vi "functiontest.vi"() -> ()   [LabVIEW 2017]
uses:
  <vilib>/regexp/Match Regular Expression.xnode
panel:
  out "trimmed string":string
  out "Commands out 2":string
  out "Commands out":string
  in  "Commands in":string
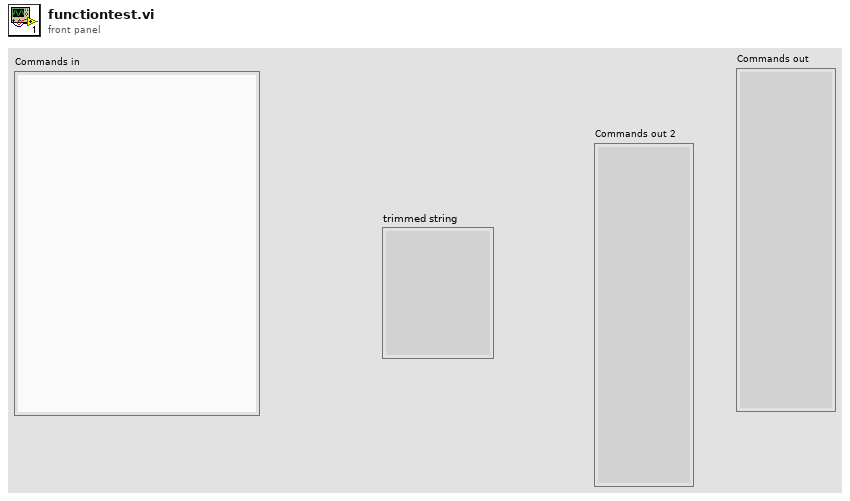
[diagram p1: front panel]
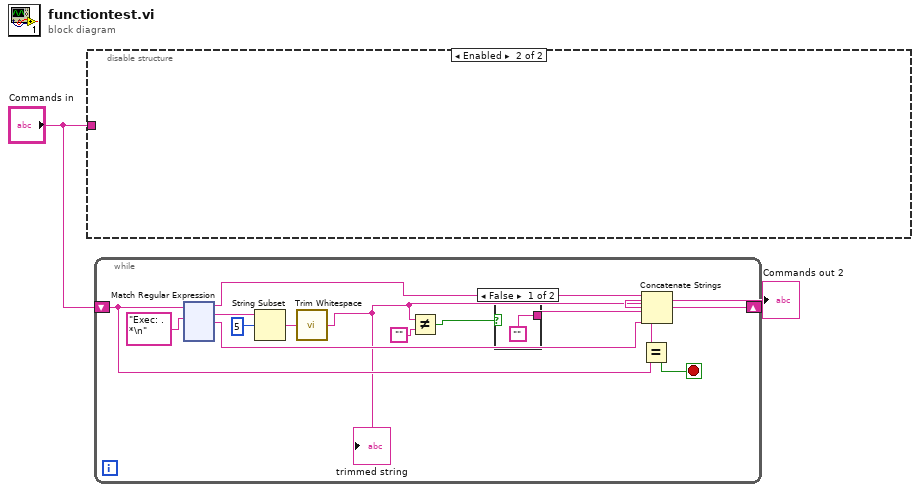
[diagram p0: block diagram]
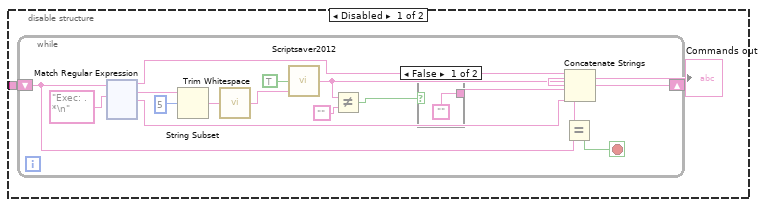
[diagram p2: hidden frame]
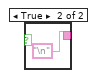
[diagram p3: hidden frame]
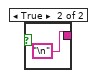
[diagram p4: hidden frame]
diagram:
  n1 = disable-structure shown="Enabled" {
    disable-tunnel: "Commands in" -> [w3 _]
    frame Disabled {
      n2 = while {
        shift-right: [w10] -> w4
        shift-left: w3 -> [w9]
        stop <- w8 stop-if-true
        n3 = xnode "Match Regular Expression"("input string"=w9, "regular expression"="Exec: .*\n") -> ("before match"=w15:string, "whole match"=w18:string, "after match"=w12:string)  [unwired: 4 in, 2 out]
        n4 = String Subset(string=w18, offset (0)=5) -> (substring=w14:string)  [unwired: 1 in]
        n5 = call <vilib>:"Trim Whitespace.vi"("string"=w14) -> ("trimmed string"=w13:string)  [unwired: 1 in]
        n6 = call "Scriptsaver2012.vi"("Filename"=w13, "Save (0)/Load (1)"=TRUE) -> ("Loaded Script"=w6:string)  [unwired: 1 in]
        n7 = Not Equal?(x=w6, y="") -> (x != y?=w5:bool)
        n8 = case shown="False" w5 {
          tunnel: ["" "\n"] -> w11
          frame False {
          }
          frame True {
          }
        }
        n9 = Concatenate Strings(w15, w6, w11, w12) -> (w10:string)
        n10 = Equal?(x=w10, y=w9) -> (x = y?=w8:bool)
      }
      "Commands out" <- w4
    }
    frame Enabled {
    }
  }
  n11 = while {
    shift-right: [w141] -> w2
    shift-left: "Commands in" -> [w140]
    stop <- w139 stop-if-true
    n12 = xnode "Match Regular Expression"("input string"=w140, "regular expression"="Exec: .*\n") -> ("before match"=w145:string, "whole match"=w147:string, "after match"=w143:string)  [unwired: 4 in, 2 out]
    n13 = String Subset(string=w147, offset (0)=5) -> (substring=w144:string)  [unwired: 1 in]
    n14 = call <vilib>:"Trim Whitespace.vi"("string"=w144) -> ("trimmed string"=w136:string)  [unwired: 1 in]
    "trimmed string" <- w136
    n15 = Not Equal?(x=w136, y="") -> (x != y?=w137:bool)
    n16 = case shown="False" w137 {
      tunnel: ["" "\n"] -> w142
      frame False {
      }
      frame True {
      }
    }
    n17 = Concatenate Strings(w145, w136, w142, w143) -> (w141:string)
    n18 = Equal?(x=w141, y=w140) -> (x = y?=w139:bool)
  }
  "Commands out 2" <- w2
